vi "PID_demo.vi"(6 "reinitialize? (F)":bool, 7 "output range":cluster{"output high":dbl, "output low":dbl}={"output high"=100.0, "output low"=-100.0} {"output low" format="%.2f"; "output high" format="%.2f"}, 8 "dt (s)":dbl=-1.0 format="%.3f", 9 "PID gains":T1={"proportional gain (Kc)"=1.0, "integral time (Ti, min)"=0.01, "derivative time (Td, min)"=0.0} {"derivative time (Td, min)" format="%.3f"; "integral time (Ti, min)" format="%.3f"; "proportional gain (Kc)" format="%.3f"}, 10 "process variable":dbl format="%.2f", 11 "setpoint":dbl format="%.2f") -> (0 "dt out (s)":dbl format="%.3f", 3 "output":dbl format="%.2f")   [LabVIEW 2010]
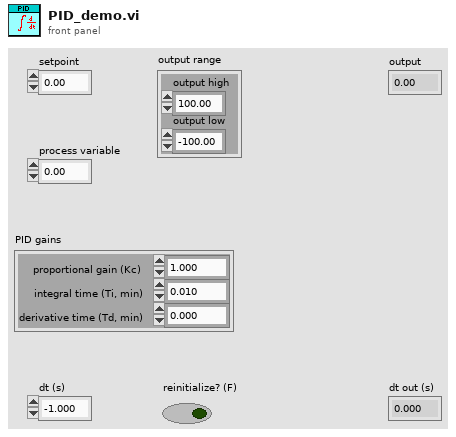
[diagram p1: front panel]
types:
  T1 = cluster{"proportional gain (Kc)":dbl, "integral time (Ti, min)":dbl, "derivative time (Td, min)":dbl}
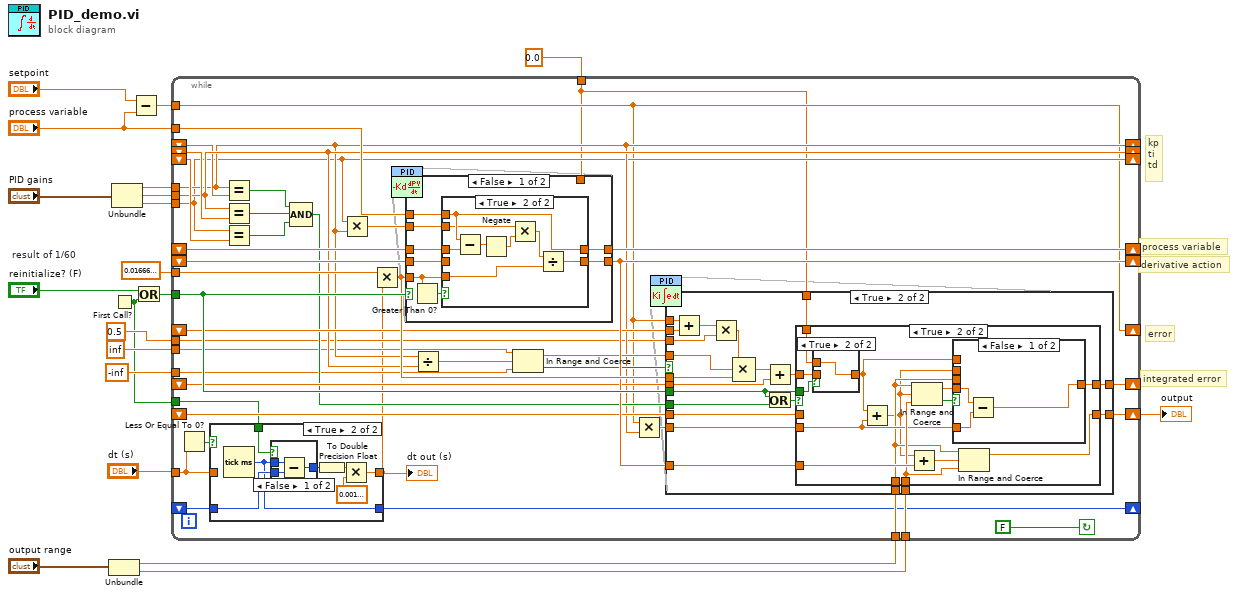
[diagram p0: block diagram]
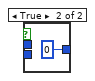
[diagram p3: hidden frame]
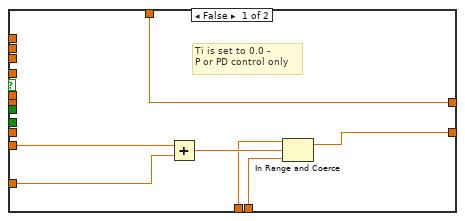
[diagram p4: hidden frame]
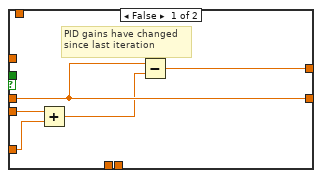
[diagram p5: hidden frame]
diagram:
  w14 = 0.016666666666666666  # result of 1/60
  # "derivative action"
  # "process variable"
  # "kp\nti\ntd"
  # "error"
  # "integrated error"
  n1 = Unbundle("output range") -> ("output high"=w16:dbl, "output low"=w15:dbl)
  n2 = First Call?() -> (First Call?: T/F=w1:bool)
  n3 = Unbundle("PID gains") -> ("proportional gain (Kc)"=w19:dbl, "integral time (Ti, min)"=w18:dbl, "derivative time (Td, min)"=w17:dbl)
  n4 = Subtract(x="setpoint", y="process variable") -> (x-y=w3:dbl)
  n5 = Or(x="reinitialize? (F)", y=w1) -> (x .or. y?=w20:bool)
  n6 = while {
    tunnel: w20 -> [w62]
    shift-left: _ -> [w24]
    shift-right: [w25] -> _
    shift-right: [w34] -> _
    shift-left: _ -> [w35]
    shift-right: [w36] -> _
    shift-left: _ -> [w59]
    shift-right: [w29] -> _
    shift-left: _ -> [w60]
    tunnel: w19 -> [w34]
    tunnel: w18 -> [w36]
    tunnel: w17 -> [w29]
    tunnel: "dt (s)" -> [w23]
    tunnel: w16 -> [w55]
    tunnel: w15 -> [w54]
    tunnel: "process variable" -> [w53]
    shift-right: [w52] -> _
    shift-left: _ -> [w51]
    shift-right: [w50] -> _
    shift-left: _ -> [w42]
    shift-right: [w49] -> w7
    shift-left: _ -> [w48]
    shift-right: [w28] -> _
    shift-left: _ -> [w47]
    shift-right: [w46] -> _
    shift-left: _ -> [w45]
    tunnel: w14 -> [w39]
    tunnel: 0.5 ("y") -> [w33]
    tunnel: inf ("upper limit") -> [w31]
    tunnel: -inf ("lower limit") -> [w32]
    tunnel: w3 -> [w28]
    tunnel: 0.0 -> [w27]
    tunnel: w1 -> [w21]
    stop <- FALSE continue-if-true
    n7 = Less Or Equal To 0?(x=w23) -> (x <= 0?=w22:bool)
    n8 = case shown="True" w22 {
      tunnel: [w64 w68] -> w26
      tunnel: w24 -> [w63 w67]
      tunnel: [w63 w66] -> w25
      tunnel: w23 -> [w64 _]
      tunnel: w21 -> [_ w65]
      frame False {
      }
      frame True {
        n9 = Tick Count (ms)() -> (millisecond timer value=w66:u32)
        n10 = case shown="False" w65 {
          tunnel: [w74 u32 0] -> w70
          tunnel: w67 -> [w73 _]
          tunnel: w66 -> [w72 _]
          frame False {
            n11 = Subtract(x=w72, y=w73) -> (x-y=w74:u32)
          }
          frame True {
          }
        }
        n12 = To Double Precision Float(number=w70) -> (double precision float=w69:dbl)
        n13 = Multiply(x=w69, y=0.0010000000474974513) -> (x*y=w68:dbl)
      }
    }
    "dt out (s)" <- w26
    n14 = Equal?(x=w34, y=w35) -> (x = y?=w57:bool)
    n15 = Equal?(x=w36, y=w59) -> (x = y?=w56:bool)
    n16 = Equal?(x=w29, y=w60) -> (x = y?=w58:bool)
    n17 = Compound Arithmetic op=AND(w57, w56, w58) -> (w37:bool)
    n18 = Multiply(x=w29, y=w34) -> (x*y=w41:dbl)
    n19 = Multiply(x=w39, y=w26) -> (x*y=w61:dbl)
    n20 = case shown="False" w62 {
      tunnel: w51 -> [w136 _]
      tunnel: w41 -> [w133 _]
      tunnel: w53 -> [w135 w148]
      tunnel: [w132 w148] -> w52
      tunnel: [w134 w147] -> w50
      tunnel: w42 -> [w130 _]
      tunnel: w61 -> [w129 _]
      tunnel: w27 -> [_ w147]
      frame False {
        n21 = Greater Than 0?(x=w129) -> (x > 0?=w131:bool)
        n22 = case shown="True" w131 {
          tunnel: w136 -> [w138 w144]
          tunnel: w129 -> [_ w143]
          tunnel: w135 -> [_ w141]
          tunnel: [w137 w142] -> w134
          tunnel: w133 -> [_ w139]
          tunnel: [w138 w141] -> w132
          tunnel: w130 -> [w137 _]
          frame False {
            # "dt = 0 min"
          }
          frame True {
            n23 = Subtract(x=w141, y=w144) -> (x-y=w146:dbl)
            n24 = Negate(x=w146) -> (-x=w140:dbl)
            n25 = Multiply(x=w139, y=w140) -> (x*y=w145:dbl)
            n26 = Divide(x=w145, y=w143) -> (x/y=w142:dbl)
          }
        }
      }
      frame True {
      }
    }
    n27 = Divide(x=w34, y=w36) -> (x/y=w40:dbl)
    n28 = In Range and Coerce(upper limit=w31, x=w40, lower limit=w32) -> (coerced(x)=w44:dbl, In Range?=w43:bool)
    n29 = Multiply(x=w28, y=w34) -> (x*y=w38:dbl)
    n30 = case shown="True" w43 {
      tunnel: w28 -> [_ w102]
      tunnel: w47 -> [_ w103]
      tunnel: w45 -> [_ w98]
      tunnel: [w76 w93] -> w46
      tunnel: w44 -> [_ w91]
      tunnel: w38 -> [w81 w96]
      tunnel: [w82 w92] -> w49
      tunnel: w48 -> [_ w94]
      tunnel: w50 -> [w80 w90]
      tunnel: w62 -> [_ w89]
      tunnel: w37 -> [_ w88]
      tunnel: w61 -> [_ w87]
      tunnel: w55 -> [w78 w85]
      tunnel: w54 -> [w77 w86]
      tunnel: w33 -> [_ w84]
      tunnel: w27 -> [w76 w83]
      frame False {
        # "Ti is set to 0.0 -\nP or PD control only"
        n31 = Add(x=w81, y=w80) -> (x+y=w79:dbl)
        n32 = In Range and Coerce(upper limit=w78, x=w79, lower limit=w77) -> (coerced(x)=w82:dbl)  [unwired: 1 out]
      }
      frame True {
        n33 = Add(x=w102, y=w103) -> (x+y=w101:dbl)
        n34 = Multiply(x=w101, y=w84) -> (x*y=w100:dbl)
        n35 = Compound Arithmetic op=MULTIPLY(w100, w91, w87) -> (w99:dbl)
        n36 = Add(x=w99, y=w98) -> (x+y=w97:dbl)
        n37 = Or(x=w89, y=w88) -> (x .or. y?=w95:bool)
        n38 = case shown="True" w95 {
          tunnel: w97 -> [_ w116]
          tunnel: w96 -> [w106 w111]
          tunnel: w94 -> [w108 _]
          tunnel: w89 -> [_ w118]
          tunnel: [w107 w113] -> w93
          tunnel: [w108 w121] -> w92
          tunnel: w90 -> [w105 w120]
          tunnel: w86 -> [_ w119]
          tunnel: w85 -> [_ w110]
          tunnel: w83 -> [_ w117]
          frame False {
            # "PID gains have changed\nsince last iteration"
            n39 = Add(x=w106, y=w105) -> (x+y=w104:dbl)
            n40 = Subtract(x=w108, y=w104) -> (x-y=w107:dbl)
          }
          frame True {
            n41 = case shown="True" w118 {
              tunnel: w117 -> [_ w128]
              tunnel: [w127 w128] -> w115
              tunnel: w116 -> [w127 _]
              frame False {
              }
              frame True {
              }
            }
            n42 = Add(x=w115, y=w111) -> (x+y=w109:dbl)
            n43 = Add(x=w109, y=w120) -> (x+y=w122:dbl)
            n44 = In Range and Coerce(upper limit=w110, x=w109, lower limit=w119) -> (coerced(x)=w112:dbl, In Range?=w114:bool)
            n45 = case shown="False" w114 {
              tunnel: w115 -> [_ w126]
              tunnel: [w123 w126] -> w113
              tunnel: w112 -> [w125 _]
              tunnel: w111 -> [w124 _]
              tunnel: w110 -> [_ _]
              tunnel: w109 -> [_ _]
              frame False {
                n46 = Subtract(x=w125, y=w124) -> (x-y=w123:dbl)
              }
              frame True {
              }
            }
            n47 = In Range and Coerce(upper limit=w110, x=w122, lower limit=w119) -> (coerced(x)=w121:dbl)  [unwired: 1 out]
          }
        }
      }
    }
  }
  "output" <- w7
